vi "RoomNumbertoIndex.vi"(8 "error in (no error)":errorcluster, 10 "y":u8, 11 "Rooms In":refnum<class "Room.lvclass">[](array[class])) -> (0 "error out":errorcluster, 1 "Room":refnum<class "Room.lvclass">, 2 "Index":i32, 3 "Rooms Out":refnum<class "Room.lvclass">[](array[class]))   [LabVIEW 2015]
uses:
  LVClasses/Room/Room.lvclass
  LVClasses/Room/Room.lvclass/Room.ctl
  LVClasses/Room/Read Room Number.vi
  <vilib>/Utility/error.llb/Error Cluster From Error Code.vi
  <vilib>/ErrorRing/Error Ring.xnode
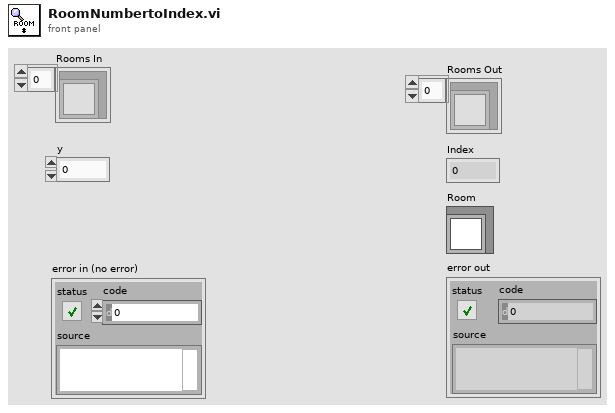
[diagram p1: front panel]
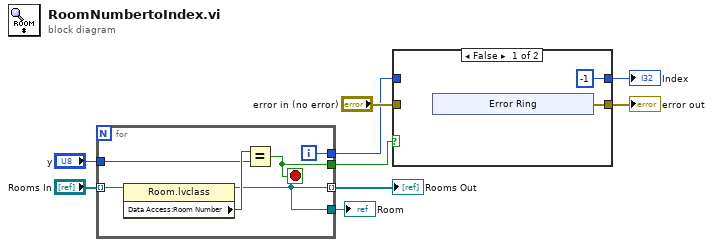
[diagram p0: block diagram]
diagram:
  n1 = for {
    tunnel: [w10] -> w9 mode=indexing
    tunnel: "Rooms In" -> [w15] mode=indexing
    tunnel: [w13] -> w4
    tunnel: [w12] -> w2
    tunnel: "y" -> [w11]
    tunnel: [w10] -> w1
    i -> [w12]
    stop <- w13 stop-if-true
    n2 = property class="Room.lvclass"(reference=w15) -> (reference out=w10:refnum<class "Room.lvclass">, "Data Access:Room Number"=w14:i32)  [unwired: 1 in, 1 out]
    n3 = Equal?(x=w14, y=w11) -> (x = y?=w13:bool)
  }
  "Rooms Out" <- w9
  "Room" <- w1
  n4 = case shown="False" w4 {
    tunnel: "error in (no error)" -> [_ w24]
    tunnel: [w17 w24] -> w5
    tunnel: [-1 ("f") w23] -> w3
    tunnel: w2 -> [_ w23]
    frame False {
      n5 = xnode "Error Ring"() -> ("error out"=w17:errorcluster)
    }
    frame True {
    }
  }
  "Index" <- w3
  "error out" <- w5
